vi "CAN Jaguar Get Transaction.vi"(8 "error in":errorcluster, 10 "Message ID":u32, 11 "CAN Jaguar Ref":T1={"Device Number"=0, "Control Mode"=enum."Percent VBus", "Inverted"=FALSE, "Semaphore"=refnum, "Max Vout"=12.0, "DevStatus"={"status"=FALSE, "code"=0, "source"=""}}) -> (0 "error out":errorcluster, 1 "Data":u8[](array[numeric]), 3 "CAN Jaguar Ref Out":T1={"Device Number"=0, "Control Mode"=enum."Percent VBus", "Inverted"=FALSE, "Semaphore"=refnum, "Max Vout"=12.0, "DevStatus"={"status"=FALSE, "code"=0, "source"=""}})   [LabVIEW 2009, in "CAN.lvlib"]
uses:
  CAN.lvlib
  CAN Jaguar Control Mode.ctl
  CAN Jaguar Ref.ctl
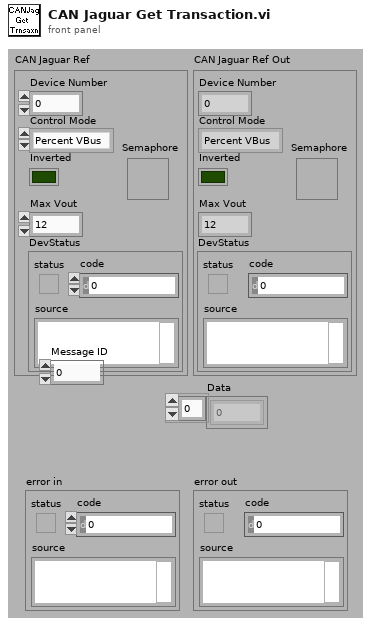
[diagram p1: front panel]
types:
  T1 = typedef "CAN.lvlib/CAN Jaguar Ref.ctl" = cluster{"Device Number":u8, "Control Mode":T2, "Inverted":bool, "Semaphore":T3, "Max Vout":dbl, "DevStatus":errorcluster}
  T2 = typedef "CAN.lvlib/CAN Jaguar Control Mode.ctl" = enum16{"Percent VBus", "Speed", "Position", "Current"}
  T3 = typedef "Semaphore RefNum" = refnum<k1>
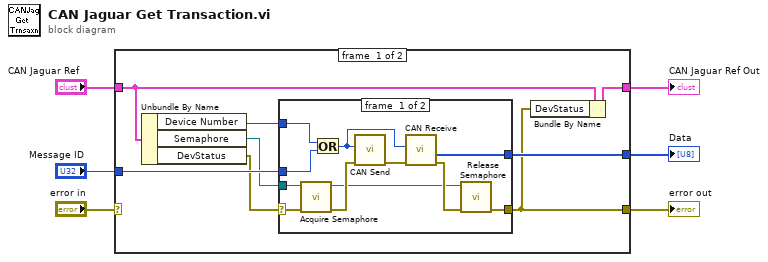
[diagram p0: block diagram]
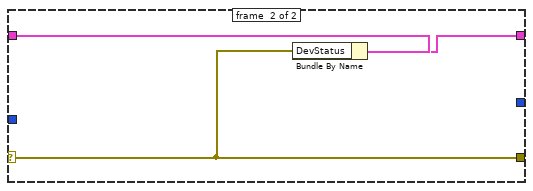
[diagram p3: hidden frame]
diagram:
  n1 = case shown="No Error" "error in" {
    selector: "error in" -> [_ w27]
    tunnel: "Message ID" -> [w14 _]
    tunnel: [w8 w27] -> w5
    tunnel: "CAN Jaguar Ref" -> [w10 w29]
    tunnel: [w13 _] -> w3
    tunnel: [w9 w28] -> w1
    frame #0 {
      n2 = Unbundle By Name(w10) -> ("Device Number"=w11:u8, "Semaphore"=w12:T3, "DevStatus"=w7:errorcluster)
      n3 = case shown="No Error" w7 {
        selector: w7 -> [w15 w26]
        tunnel: w14 -> [w24 _]
        tunnel: [w22 _] -> w13
        tunnel: w12 -> [w21 _]
        tunnel: w11 -> [w19 _]
        tunnel: [w17 w26] -> w8
        frame #0 {
          n4 = call <vilib>:"Acquire Semaphore.vi"("error in (no error)"=w15, "semaphore"=w21) -> ("error out"=w20:errorcluster, "semaphore out"=w16:T3)  [unwired: 1 in, 3 out]
          n5 = Or(x=w19, y=w24) -> (x .or. y?=w23:u32)
          n6 = call "CAN Send.vi"("error in (no error)"=w20, "messageID"=w23) -> ("error out"=w25:errorcluster)  [unwired: 1 in, 8 out]
          n7 = call "CAN Receive.vi"("error in (no error)"=w25, "Message ID"=w23) -> ("error out"=w18:errorcluster, "data"=w22:u8[])  [unwired: 1 in, 7 out]
          n8 = call <vilib>:"Release Semaphore.vi"("error in (no error)"=w18, "semaphore"=w16) -> ("error out"=w17:errorcluster)  [unwired: 5 out]
        }
        frame #1 {
        }
      }
      n9 = Bundle By Name(cluster=w10, "DevStatus"=w8) -> (w9:T1)
    }
    frame #1 {
      n10 = Bundle By Name(cluster=w29, "DevStatus"=w27) -> (w28:T1)
    }
  }
  "Data" <- w3
  "error out" <- w5
  "CAN Jaguar Ref Out" <- w1
